vi "Add additional rows to command file.vi"(1 "Table In":T1[](array[typedef]) {"Carrier_2 Q (l/min)" format="%#.2f"; "Row Duration (mins)" format="%#.1f"; "Row No" min=0; "Trace Gas Concentration (%)" min=0.0 format="%#_4f"; "Carrier_1 Q (l/min)" format="%#.4f"; "Start X" format="%#.2f"; "Start Y" format="%#.2f"; "Start Z" format="%#.2f"; "End X" format="%#.2f"; "End Y" format="%#.2f"; "End Z" format="%#.2f"; "Tunnel Speed" format="%#.2f"; "Averaging time (mins)" min=0.0 format="%#.2f"}) -> (0 "Table Out":T1[](array[typedef]) {"Carrier_2 Q (l/min)" format="%#.2f"; "Row Duration (mins)" format="%#.1f"; "Row No" min=0; "Trace Gas Concentration (%)" min=0.0 format="%#_4f"; "Carrier_1 Q (l/min)" format="%#.4f"; "Start X" format="%#.2f"; "Start Y" format="%#.2f"; "Start Z" format="%#.2f"; "End X" format="%#.2f"; "End Y" format="%#.2f"; "End Z" format="%#.2f"; "Tunnel Speed" format="%#.2f"; "Averaging time (mins)" min=0.0 format="%#.2f"})   [LabVIEW 2022 SP3]
uses:
  Traverse_cluster.ctl
  Spacing.ctl
  Controls/Multi_run_mode.ctl
  <vilib>/Utility/error.llb/Trim Whitespace One-Sided.vi
panel:
  # "X           Y          Z"
  # "Start"
  # "End"
  # "X           Y          Z"
  # "Start"
  # "End"
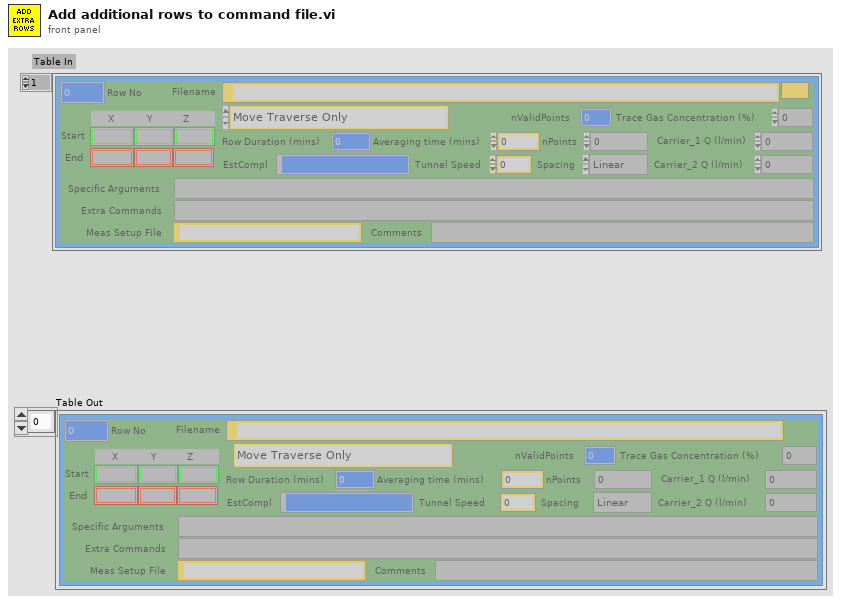
[diagram p1: front panel]
types:
  T1 = typedef "Traverse_cluster.ctl" = cluster{"Start X":sgl, "Start Y":sgl, "Start Z":sgl, "End X":sgl, "End Y":sgl, "End Z":sgl, "nPoints":i32, "Spacing":T2, "Filename":path, "Tunnel Speed":dbl, "Averaging time (mins)":dbl, "Extra Commands":string, "Carrier_1 Q (l/min)":dbl, "Carrier_2 Q (l/min)":dbl, "Trace Gas Concentration (%)":dbl, "Specific Arguments":string, "Comments":string, "Row No":i32, "Row Type Selector":T3, "EstCompl":string, "Row Duration (mins)":dbl, "nValidPoints":i32, "Meas Setup File":string}
  T2 = typedef "Spacing.ctl" = enum16{"Linear", "Log", "Gauss", "Specified", "N/A"}
  T3 = typedef "Multi_run_mode.ctl" = enum16{"Move Traverse Only", "Set Tunnel Speed Only", "Set Source Only", "Set Measurement Conditions", "Single Measurement", "Vertical Profile", "Lateral Profile", "Longitudinal Profile", "Multi-Axis Profile", "Explore Volume", "Auto Calibrate", "Meas Fast FID Bkgnd", "Check Beam Power", "Scanning Valve Measurement", "Run VI Named:", "Set ADAM Ch", "Wait (minutes)", "Send Message", "Synchronize With:", "Fall Back to this Row", "Turn Off Row Repeating", "Traverse 3D Volume", "Blank Row", "Jump to Fall Back Row"}
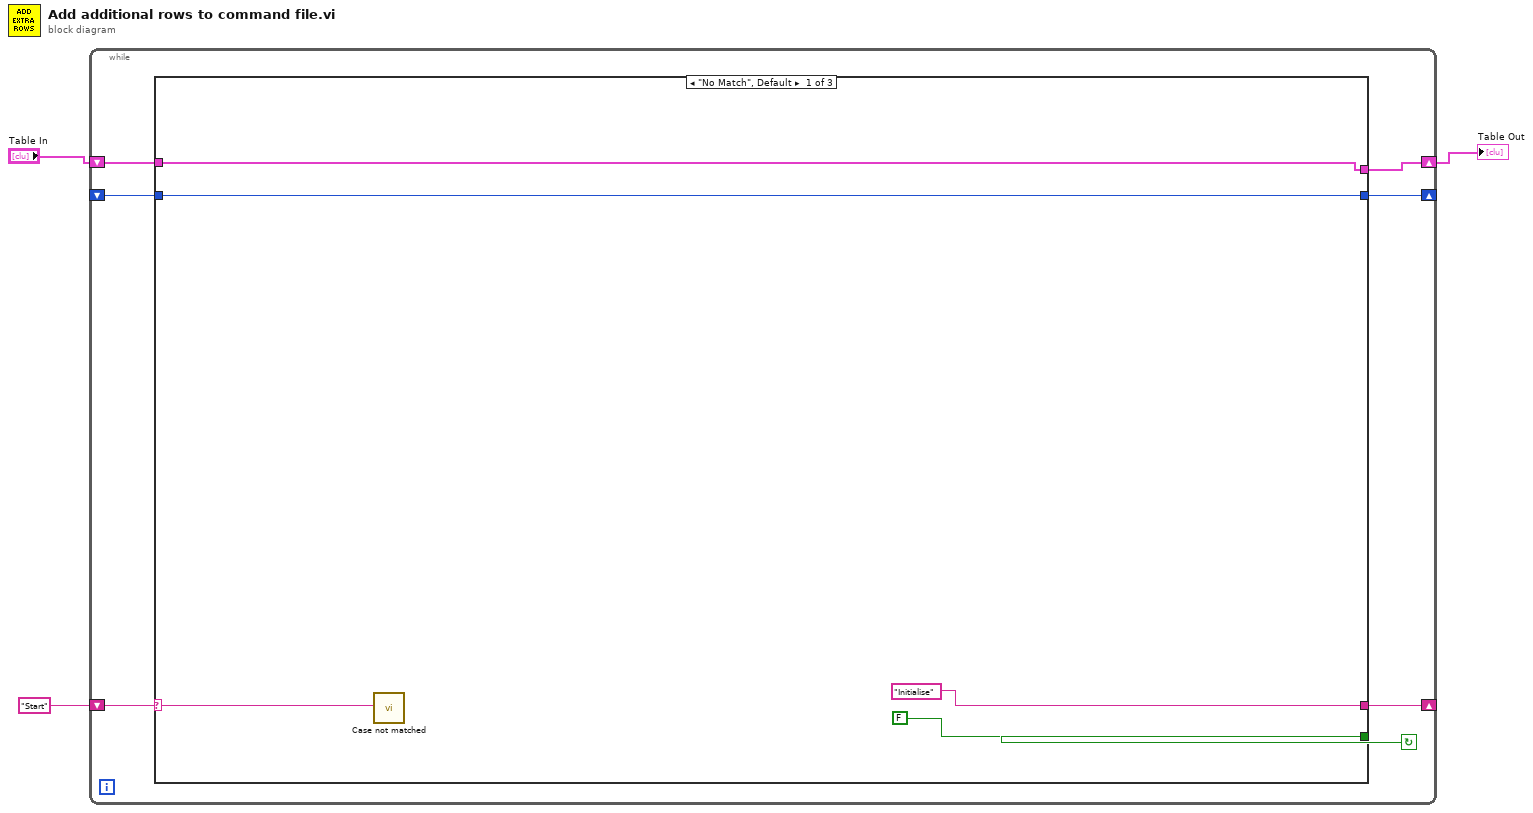
[diagram p0: block diagram]
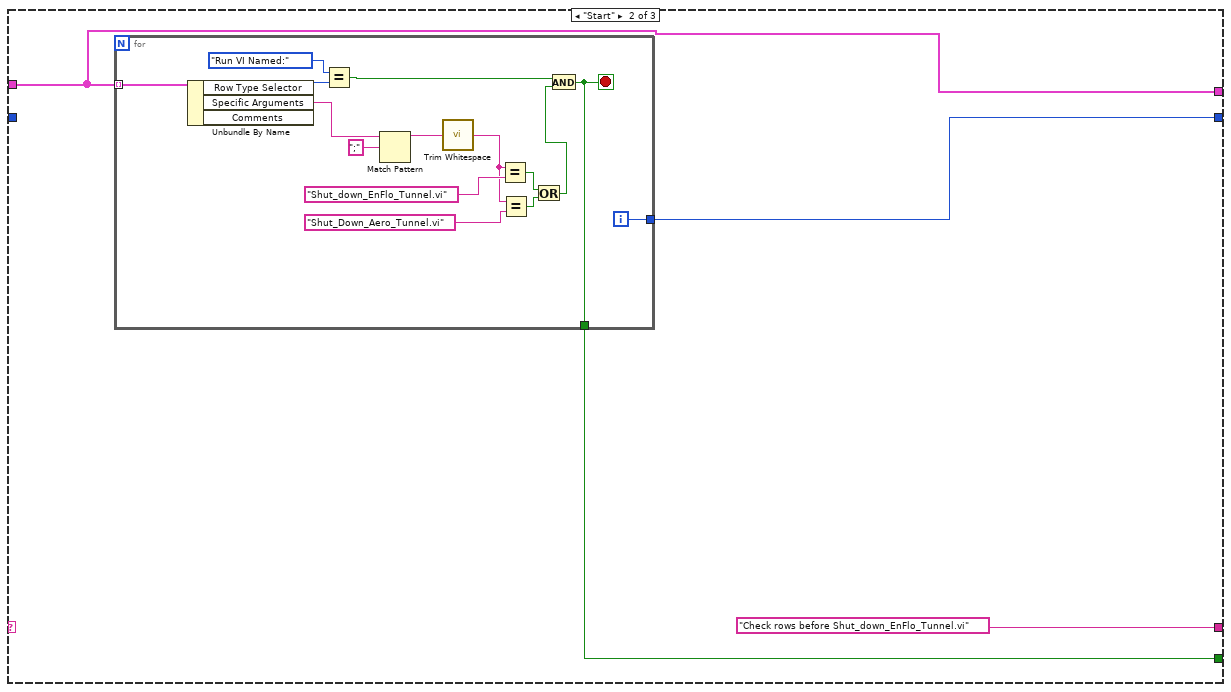
[diagram p2: hidden frame]
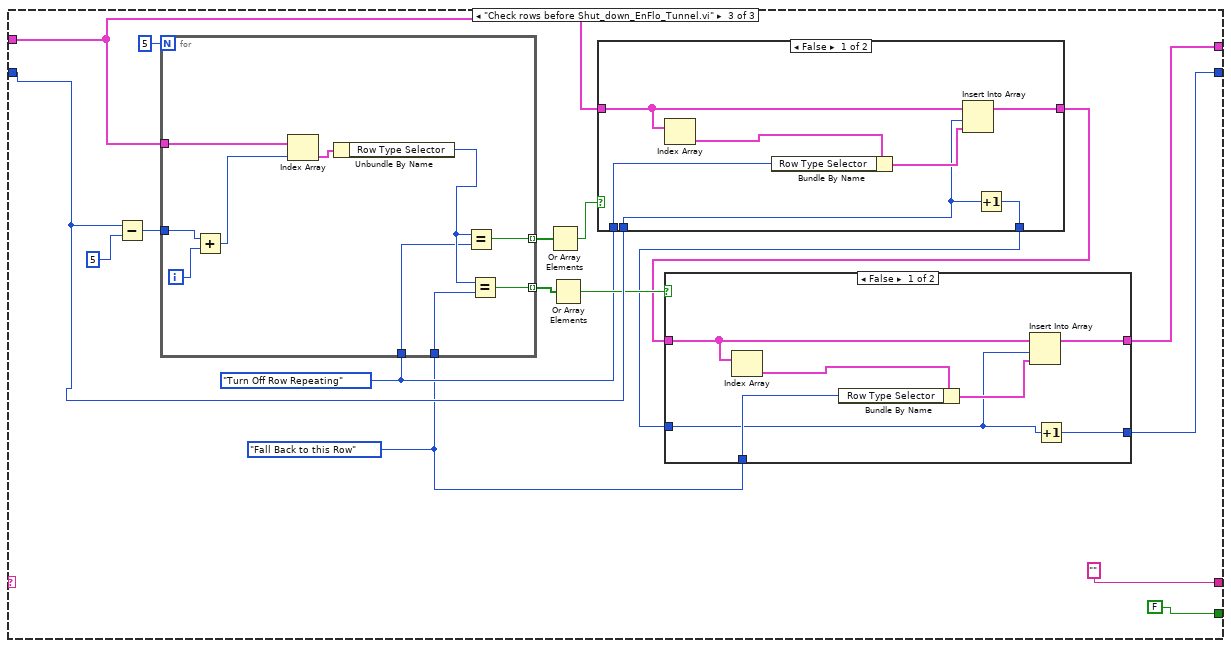
[diagram p3: hidden frame]
diagram:
  n1 = while {
    shift-left: "Start" -> [w8]
    shift-right: [w9] -> _
    shift-right: [w5] -> w1
    shift-left: "Table In" -> [w7]
    shift-right: [w6] -> _
    shift-left: _ -> [w4]
    stop <- w10 continue-if-true
    n2 = case shown="\"No Match\", Default" w8 {
      selector: w8 -> [w11 _ _]
      tunnel: [FALSE w18 FALSE] -> w10
      tunnel: ["Initialise" "Check rows before Shut_down_EnFlo_Tunnel.vi" ""] -> w9
      tunnel: w7 -> [w13 w16 w43]
      tunnel: [w12 w17 w35] -> w6
      tunnel: [w13 w16 w36] -> w5
      tunnel: w4 -> [w12 _ w44]
      frame "No Match", Default {
        n3 = call "Case not matched.vi"("Case Name not Matched"=w11) -> ()
      }
      frame "Start" {
        n4 = for {
          tunnel: w16 -> [w34] mode=indexing
          tunnel: [w27] -> w18
          tunnel: [w26] -> w17
          i -> [w26]
          stop <- w27 stop-if-true
          n5 = Unbundle By Name(w34) -> ("Row Type Selector"=w25:T3, "Specific Arguments"=w30:string)  [unwired: 1 out]
          n6 = Equal?(x=Multi_run_mode."Run VI Named:" ("Row Type Selector"), y=w25) -> (x = y?=w28:bool)
          n7 = Match Pattern(string=w30, regular expression=";") -> (before substring=w31:string)  [unwired: 4 out]
          n8 = call <vilib>:"Trim Whitespace.vi"("string"=w31) -> ("trimmed string"=w24:string)  [unwired: 1 in]
          n9 = Equal?(x=w24, y="Shut_down_EnFlo_Tunnel.vi") -> (x = y?=w21:bool)
          n10 = Equal?(x=w24, y="Shut_Down_Aero_Tunnel.vi") -> (x = y?=w22:bool)
          n11 = Or(x=w21, y=w22) -> (x .or. y?=w20:bool)
          n12 = And(x=w28, y=w20) -> (x .and. y?=w27:bool)
        }
      }
      frame "Check rows before Shut_down_EnFlo_Tunnel.vi" {
        w37 = Multi_run_mode."Fall Back to this Row" ("Row Type Selector")
        w38 = Multi_run_mode."Turn Off Row Repeating" ("Row Type Selector")
        n13 = Subtract(x=w44, y=5) -> (x-y=w47:i32)
        n14 = for {
          N: 5 -> [_]
          tunnel: w43 -> [w78]
          tunnel: w47 -> [w76]
          tunnel: [w73] -> w46 mode=indexing
          tunnel: [w72] -> w42 mode=indexing
          tunnel: w38 -> [w71]
          tunnel: w37 -> [w70]
          i -> [w77]
          n15 = Add(x=w76, y=w77) -> (x+y=w75:i32)
          n16 = Index Array(array=w78, index=w75) -> (element=w74:T1)
          n17 = Unbundle By Name(w74) -> ("Row Type Selector"=w79:T3)
          n18 = Equal?(x=w79, y=w71) -> (x = y?=w73:bool)
          n19 = Equal?(x=w79, y=w70) -> (x = y?=w72:bool)
        }
        n20 = Or Array Elements(Boolean array=w46) -> (logical OR=w45:bool)
        n21 = Or Array Elements(Boolean array=w42) -> (logical OR=w41:bool)
        n22 = case shown="False" w45 {
          tunnel: w44 -> [w63 w69]
          tunnel: w43 -> [w67 w68]
          tunnel: [w64 w68] -> w39
          tunnel: [w62 w69] -> w40
          tunnel: w38 -> [w61 _]
          frame False {
            n23 = Index Array(array=w67) -> (element=w66:T1)  [unwired: 1 in]
            n24 = Bundle By Name(cluster=w66, "Row Type Selector"=w61) -> (w65:T1)
            n25 = Insert Into Array(array=w67, index=w63, new element=w65) -> (w64:T1[])
            n26 = Increment(x=w63) -> (x+1=w62:i32)
          }
          frame True {
          }
        }
        n27 = case shown="False" w41 {
          tunnel: w39 -> [w58 w60]
          tunnel: [w55 w60] -> w36
          tunnel: w40 -> [w53 w59]
          tunnel: w37 -> [w54 _]
          tunnel: [w52 w59] -> w35
          frame False {
            n28 = Index Array(array=w58) -> (element=w57:T1)  [unwired: 1 in]
            n29 = Bundle By Name(cluster=w57, "Row Type Selector"=w54) -> (w56:T1)
            n30 = Insert Into Array(array=w58, index=w53, new element=w56) -> (w55:T1[])
            n31 = Increment(x=w53) -> (x+1=w52:i32)
          }
          frame True {
          }
        }
      }
    }
  }
  "Table Out" <- w1
